vi "busy_wait_embed.vi"(7 "caller":refnum<vi>, 8 "error in (no error)":errorcluster, 11 "configuration":T2={"dialog_text"="", "wait_s"=0.0, "inner_color"=16711680, "outer_color"=6618880, "knob_reference"=refnum, "dialog_reference"=refnum, "event_registration"=refnum}) -> (0 "error out":errorcluster, 3 "dialog_selection":T1)   [LabVIEW 2015, in "lv-dialog-interfaces.lvlib"]
uses:
  lv-dialog-interfaces.lvlib
  <userlib>/antonio-alexander/lv-dialog/api/v1/public/_controls/selection.ctl
  private/_controls/dialog_type.ctl
  private/_controls/hmi_references.ctl
  private/_controls/configuration.ctl
  <userlib>/antonio-alexander/lv-dialog/api/v1/v1.lvlib
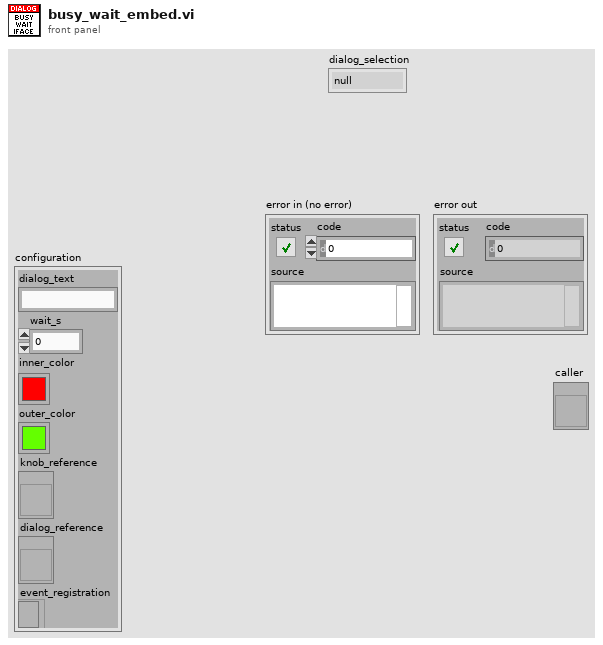
[diagram p1: front panel]
types:
  T1 = typedef "lv-dialog.lvlib/v1.lvlib/selection.ctl" = enum16{"null", "panel_closed", "button_1", "button_2", "button_3", "cancelled"}
  T2 = cluster{"dialog_text":string, "wait_s":dbl, "inner_color":u32, "outer_color":u32, "knob_reference":refnum<vi>, "dialog_reference":refnum<vi>, "event_registration":refnum<event-registration>}
  T3 = typedef "lv-dialog-interfaces.lvlib/dialog_type.ctl" = enum16{"null", "one_button", "two_button", "three_button", "confirmation", "busy_wait", "error", "busy_wait_embed", "combo_box", "data_entry_string", "data_entry_numeric"}
  T4 = typedef "lv-dialog-interfaces.lvlib/configuration.ctl" = cluster{"dialog_text":string, "boolean_text_1":string, "boolean_text_2":string, "boolean_text_3":string, "inner_color":u32, "outer_color":u32, "wait_s":dbl, "error_status":bool, "error_source":string, "error_details":string, "string []":string[], "custom_entry":bool, "confirmation_text":string}
  T5 = typedef "lv-dialog-interfaces.lvlib/hmi_references.ctl" = cluster{"vi_reference":refnum<vi>, "caller":refnum<vi>, "dialog":refnum<vi>, "button_1":refnum<vi>, "button_2":refnum<vi>, "button_3":refnum<vi>, "busy":refnum<vi>, "error_glyph":refnum<vi>, "error_source":refnum<vi>, "error_text":refnum<vi>, "combo_box":refnum<vi>}
  T6 = cluster{"dialog_text":string, "boolean_text_1":string, "boolean_text_2":string}
  T7 = cluster{"dialog_text":string, "boolean_text_1":string}
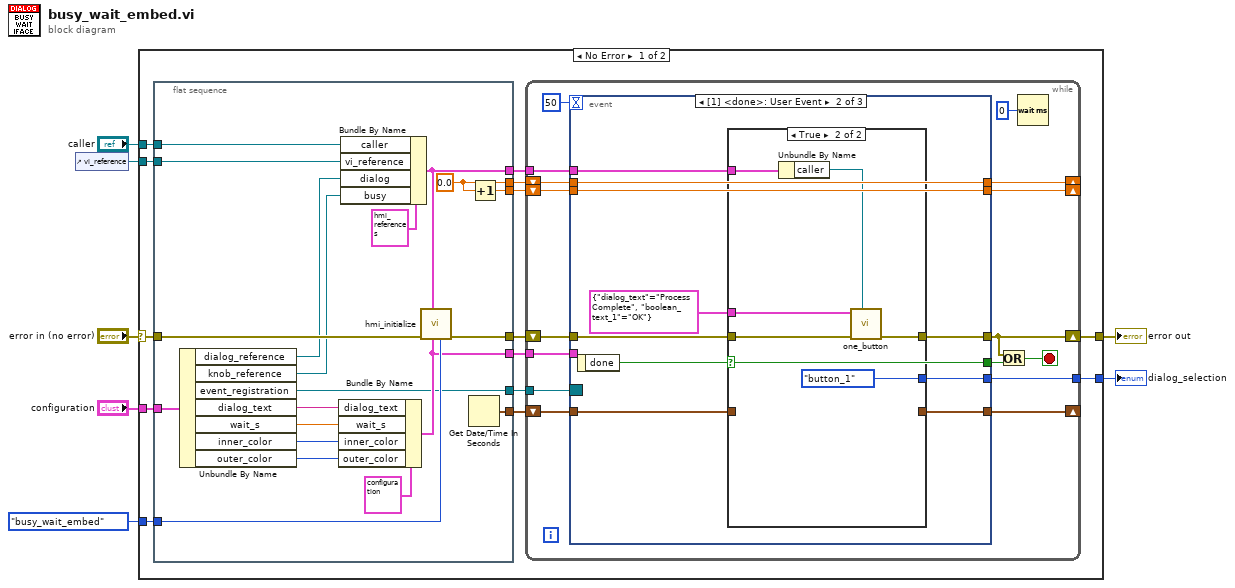
[diagram p0: block diagram]
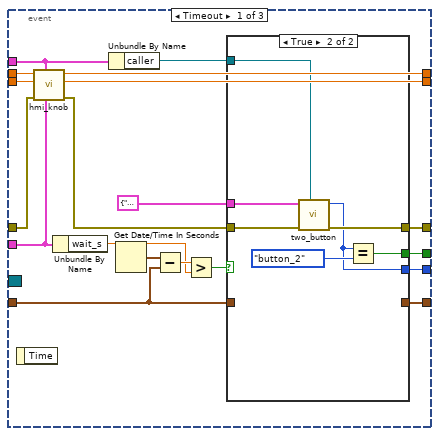
[diagram p2: hidden frame]
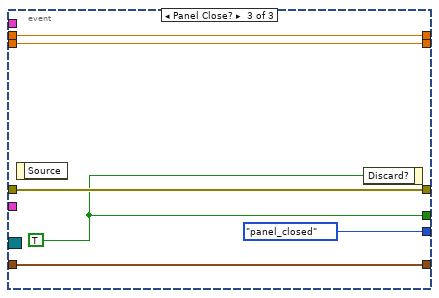
[diagram p5: hidden frame]
diagram:
  n1 = control-ref of="vi_reference"() -> (w3:refnum<vi>)
  n2 = case shown="No Error" "error in (no error)" {
    selector: "error in (no error)" -> [w21 w110]
    tunnel: "caller" -> [w20 _]
    tunnel: "configuration" -> [w19 _]
    tunnel: dialog_type."busy_wait_embed" ("dialog_type") -> [w18 _]
    tunnel: [w8 w110] -> w4
    tunnel: w3 -> [w12 _]
    tunnel: [w11 _] -> w1
    frame No Error {
      n3 = flat-sequence {
        tunnel: [w41] -> w17
        tunnel: [w40] -> w16
        tunnel: [w34] -> w9
        tunnel: w21 -> [w39]
        tunnel: [w36] -> w15
        tunnel: [w35] -> w14
        tunnel: w19 -> [w30]
        tunnel: [w31] -> w13
        tunnel: w20 -> [w33]
        tunnel: w18 -> [w37]
        tunnel: w12 -> [w24]
        tunnel: [w22] -> w10
        frame #0 {
          w35 = 0.0
          n4 = Unbundle By Name(w30) -> ("dialog_reference"=w23:refnum<vi>, "knob_reference"=w25:refnum<vi>, "event_registration"=w22:refnum<event-registration>, "dialog_text"=w29:string, "wait_s"=w28:dbl, "inner_color"=w27:u32, "outer_color"=w26:u32)
          n5 = Bundle By Name(cluster=T4 {"dialog_text"="", "boolean_text_1"="", "boolean_text_2"="", "boolean_text_3"="", "inner_color"=16711680, "outer_color"=6618880, "wait_s"=nan, "error_status"=FALSE, "error_source"="", "error_details"="", "string []"=[], "custom_entry"=FALSE, "confirmation_text"=""} ("configuration"), "dialog_text"=w29, "wait_s"=w28, "inner_color"=w27, "outer_color"=w26) -> (w31:T4)
          n6 = Bundle By Name(cluster=T5 {"vi_reference"=refnum, "caller"=refnum, "dialog"=refnum, "button_1"=refnum, "button_2"=refnum, "button_3"=refnum, "busy"=refnum, "error_glyph"=refnum, "error_source"=refnum, "error_text"=refnum, "combo_box"=refnum} ("references"), "caller"=w33, "vi_reference"=w24, "dialog"=w23, "busy"=w25) -> (w34:T5)
          n7 = call "hmi_initialize.vi"("dialog_type"=w37, "configuration"=w31, "references"=w34, "error in (no error)"=w39) -> ("error out"=w36:errorcluster)  [unwired: 7 in]
          n8 = Get Date/Time In Seconds() -> (seconds since 1Jan1904=w40:timestamp)
          n9 = Increment(x=w35) -> (x+1=w41:dbl)
        }
      }
      n10 = while {
        shift-right: [w57] -> _
        shift-left: w14 -> [w54]
        shift-right: [w56] -> _
        shift-left: w17 -> [w55]
        shift-right: [w44] -> w8
        shift-left: w15 -> [w53]
        shift-right: [w49] -> _
        shift-left: w16 -> [w50]
        tunnel: w13 -> [w48]
        tunnel: [w43] -> w11
        tunnel: w10 -> [w42]
        tunnel: w9 -> [w47]
        stop <- w45 stop-if-true
        n11 = event shown="[1] <done>: User Event" {
          selector: w42 -> [_ _ _]
          dyn-events: _ -> [_ _ _]
          timeout: 50 -> [_ _ _]
          tunnel: [w70 w95 w108] -> w57
          tunnel: [w71 w94 w107] -> w56
          tunnel: w55 -> [w69 w94 w107]
          tunnel: w54 -> [w68 w95 w108]
          tunnel: w53 -> [w76 w92 w109]
          tunnel: [w72 w91 w109] -> w44
          tunnel: [w63 w86 w106] -> w46
          tunnel: w50 -> [w59 w88 w105]
          tunnel: [w58 w87 w105] -> w49
          tunnel: w48 -> [w66 _ _]
          tunnel: w47 -> [w65 w90 _]
          tunnel: [w61 w89 selection."panel_closed" ("dialog_selection")] -> w43
          event Timeout {
            n12 = event-data() -> ()  [unwired: 1 in, 1 out]
            n13 = call "hmi_knob.vi"("configuration"=w66, "hmi_references"=w65, "error in (no error)"=w76, "value_2 in"=w69, "value_1 in"=w68) -> ("error out"=w73:errorcluster, "value_2 out"=w71:dbl, "value_1 out"=w70:dbl)  [unwired: 4 in]
            n14 = Unbundle By Name(w66) -> ("wait_s"=w67:dbl)
            n15 = Unbundle By Name(w65) -> ("caller"=w64:refnum<vi>)
            n16 = Get Date/Time In Seconds() -> (seconds since 1Jan1904=w75:timestamp)
            n17 = Subtract(x=w75, y=w59) -> (x-y=w74:dbl)
            n18 = Greater?(x=w74, y=w67) -> (0:w60:bool)
            n19 = case shown="True" w60 {
              tunnel: w73 -> [w78 w83]
              tunnel: [w78 w82] -> w72
              tunnel: [_ w84] -> w63
              tunnel: w64 -> [_ w81]
              tunnel: T6 {"dialog_text"="Waiting process has not completed.", "boolean_text_1"="Wait", "boolean_text_2"="Continue"} -> [_ w80]
              tunnel: [_ w79] -> w61
              tunnel: w59 -> [w77 _]
              tunnel: [w77 _] -> w58
              frame False {
              }
              frame True {
                n20 = call "two_button.vi"("callee"=w81, "error in (no error)"=w83, "configuration"=w80) -> ("error out"=w82:errorcluster, "dialog_selection"=w79:T1)  [unwired: 7 in]
                n21 = Equal?(x=w79, y=selection."button_2" ("x")) -> (x = y?=w84:bool)
              }
            }
          }
          event User Event {
            n22 = event-data() -> ("done"=w86:bool)  [unwired: 1 in]
            n23 = case shown="True" w86 {
              tunnel: w92 -> [w97 w103]
              tunnel: [w97 w102] -> w91
              tunnel: w90 -> [_ w101]
              tunnel: T7 {"dialog_text"="Process Complete", "boolean_text_1"="OK"} ("configuration") -> [_ w99]
              tunnel: [_ selection."button_1" ("dialog_selection")] -> w89
              tunnel: w88 -> [w96 _]
              tunnel: [w96 _] -> w87
              frame False {
              }
              frame True {
                n24 = Unbundle By Name(w101) -> ("caller"=w100:refnum<vi>)
                n25 = call "one_button.vi"("callee"=w100, "error in (no error)"=w103, "configuration"=w99) -> ("error out"=w102:errorcluster)  [unwired: 7 in, 1 out]
              }
            }
          }
          event Panel Close? {
            w106 = TRUE
            n26 = event-data() -> ()  [unwired: 1 in, 1 out]
            n27 = event-data("Discard?"=w106) -> ()  [unwired: 1 in, 1 out]
          }
        }
        n28 = Or(x=w44, y=w46) -> (x .or. y?=w45:bool)
        n29 = Wait (ms)(milliseconds to wait=u32 0) -> ()  [unwired: 1 out]
      }
    }
    frame Error {
    }
  }
  "error out" <- w4
  "dialog_selection" <- w1
